vi "Create_Results_Row.vi"() -> (0 "row splitting":string[][](array[string]), 1 "Channel Values":string[](array[string]), 2 "Channel Names":string[](array[string]))   [LabVIEW 2012]
uses:
  Globals/Meas_global.vi
  Globals/Trav_pos_global.vi
  Globals/Dynamic_call_global.ph.vi
  Globals/LDA_meas_global_1.vi
  Acquisition/PWA/PWAtasksGLOBAL.vi
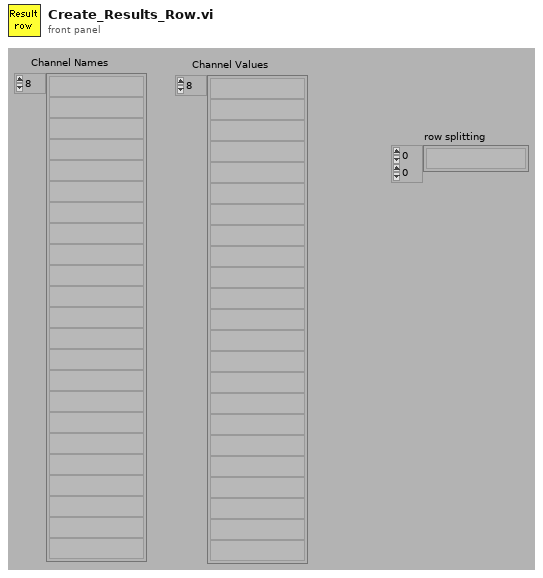
[diagram p1: front panel]
types:
  T1 = typedef "Analysis_info_cluster.ctl" = cluster{"Colour":u32, "Inst type":T2, "Inst name":string, "Symbol":string, "Code name":string, "Extra Info":string, "Inst Array":T3, "Extra Titles":string[], "Extra Values":string[], "U":dbl, "u^2":dbl, "u^3":dbl, "u^4":dbl, "Skew_u":dbl, "Kurt_u":dbl, "Sd Error in Mean":dbl, "% u'/U":dbl, "X":dbl, "Y":dbl, "Z":dbl, "Timescale integral to 25%":dbl, "Sd Error in Variance":dbl, "Calib File":path, "Calib Constants":dbl[], "Output Position":bool, "Full Stats":bool, "Av Sampling Rate":dbl, "Av No of Samples":dbl, "Total Meas Time (s)":dbl, "ADAM Ch Name":string}
  T2 = typedef "Inst_type.ctl" = enum16{"Propeller anemometer", "Raw voltage", "Pressure Transducer", "Pitot-static tube", "Preston tube", "Hot wire", "Cross wire 1", "Cross wire 2", "Generic Linear", "Generic Polynomial", "Generic BackPoly", "Fast FID", "Thermocouple", "Cold wire", "Pulsed Wire", "LDA Vel", "LDA Tran time", "LDA Arr time"}
  T3 = typedef "Instrument_Array.ctl" = enum16{"PWA", "LDA", "Analogue"}
  T4 = typedef "Post_Process.ctl" = enum16{"Take New Data", "Post Process Raw Data File"}
  T5 = typedef "PWA_Data.ctl" = enum16{"No PWA Data", "One Ch PWA"}
  T6 = typedef "Correlation_cluster1.ctl" = cluster{"U inst":string, "uw":dbl, "u^2w":dbl, "uw^2":dbl, "uw/u'w'":dbl, "W inst":string, "uw^3":dbl, "u^3w":dbl, "u^2w^2":dbl, "Index U":i32, "Index W":i32}
  T7 = typedef "Traverse_cluster.ctl" = cluster{"Start X":dbl, "Start Y":dbl, "Start Z":dbl, "End X":dbl, "End Y":dbl, "End Z":dbl, "No. of pts.":i32, "Spacing":T8, "Filename":path, "Tunnel Speed":dbl, "Averaging time (min)":dbl, "Extra Commands":string, "Specific Arguments":string, "Emission Rate (l/min)":dbl, "Trace Gas Concentration (%)":dbl, "Density Ratio":string, "Comments":string, "Row No":i32, "Row Type Selector":T9, "Completion time":string, "Row Duration (mins)":dbl, "No. of Valid pts.":i32, "Meas Setup File":string}
  T8 = typedef "Spacing.ctl" = enum16{"Linear", "Log", "Gauss", "Specified", "N/A"}
  T9 = typedef "Multi_run_mode.ctl" = enum16{"Move Traverse Only", "Set Tunnel Speed Only", "Set Source Only", "Set Measurement Conditions", "Single Measurement", "Vertical Profile", "Lateral Profile", "Longitudinal Profile", "Explore Volume", "Multi-Axis Profile", "Auto Calibrate", "Meas Fast FID Bkgnd", "Check Beam Power", "Scanning Valve Measurement", "Run VI Named:", "Set ADAM Ch", "Wait (minutes)", "Send Message", "Synchronize With:", "Fall Back to this Row", "Turn Off Row Repeating", "Blank Row", "Traverse 3D Volume"}
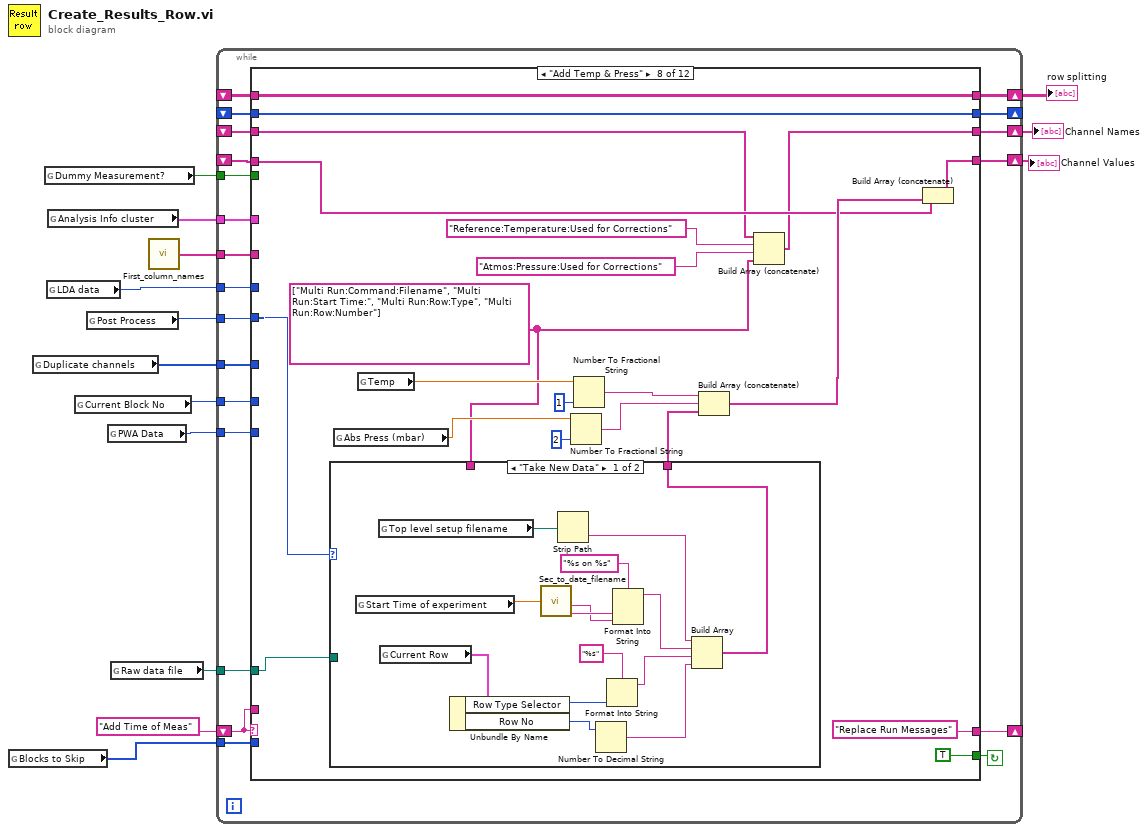
[diagram p0: block diagram]
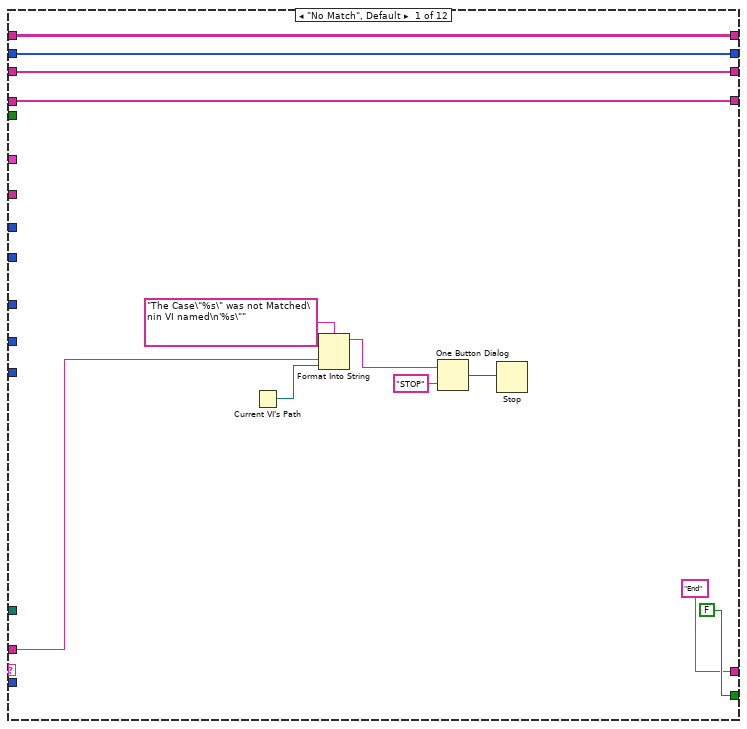
[diagram p2: hidden frame]
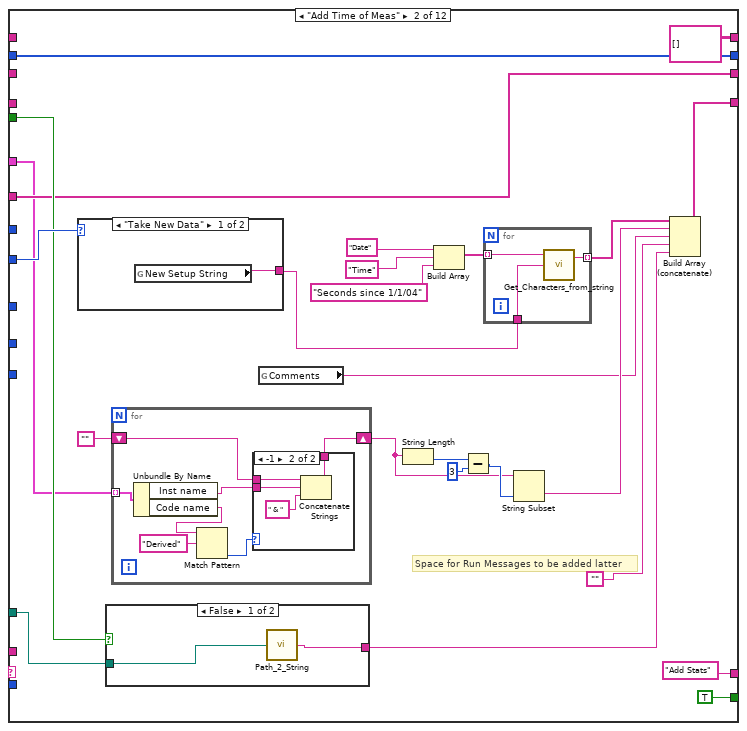
[diagram p3: hidden frame]
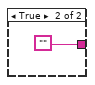
[diagram p4: hidden frame]
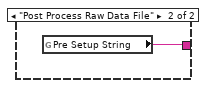
[diagram p6: hidden frame]
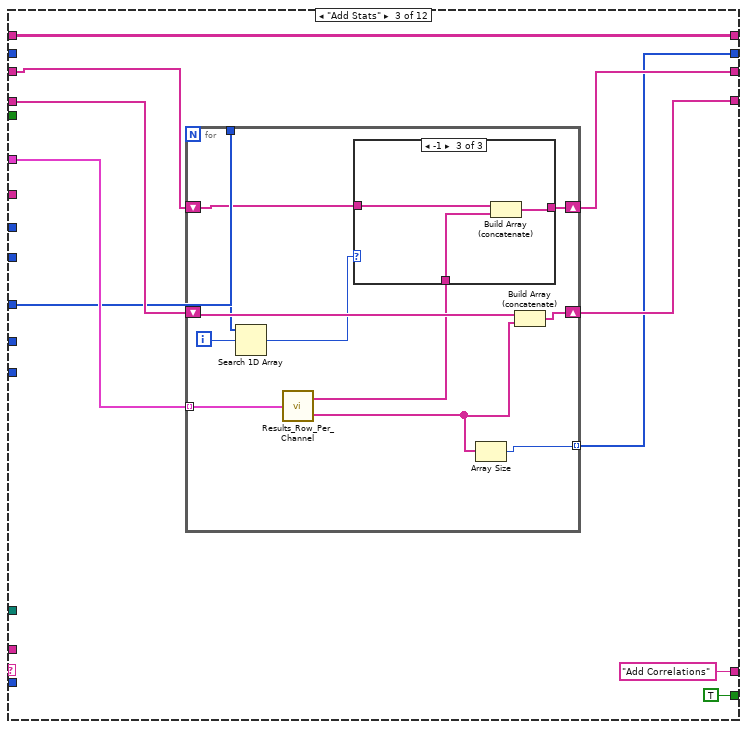
[diagram p7: hidden frame]
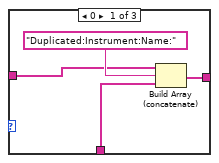
[diagram p8: hidden frame]
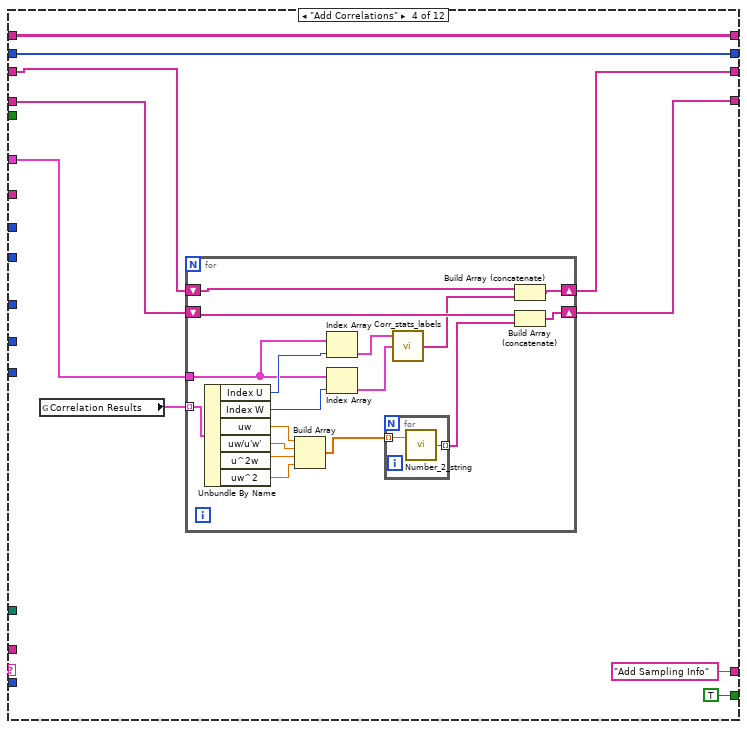
[diagram p10: hidden frame]
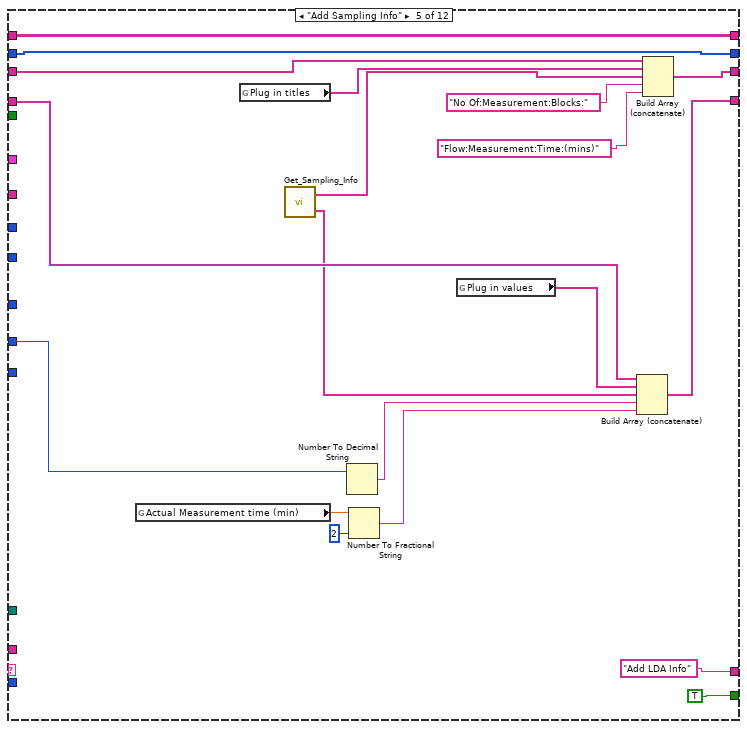
[diagram p11: hidden frame]
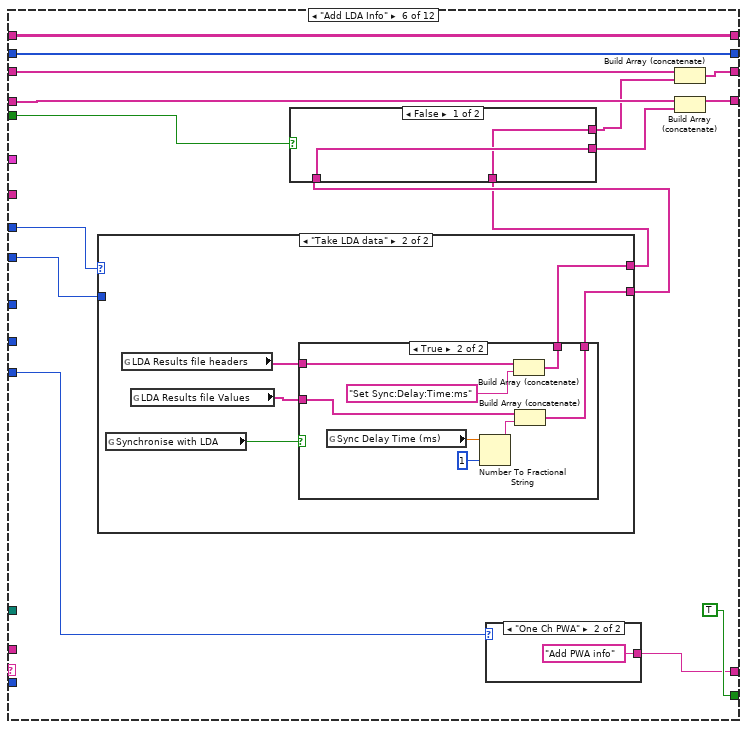
[diagram p12: hidden frame]
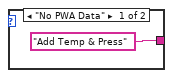
[diagram p13: hidden frame]
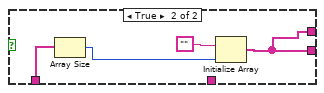
[diagram p14: hidden frame]
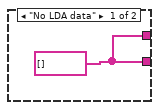
[diagram p15: hidden frame]
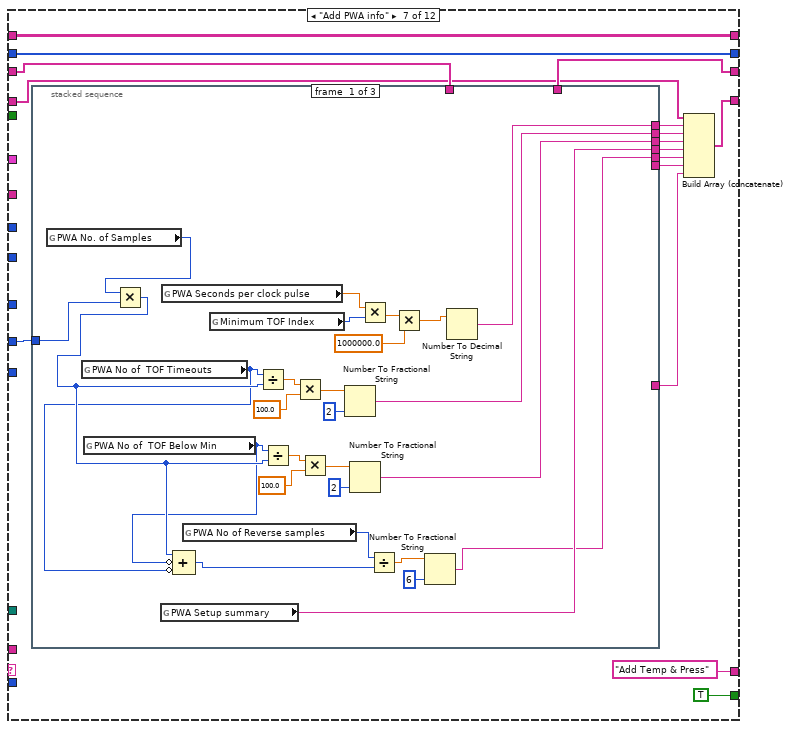
[diagram p17: hidden frame]
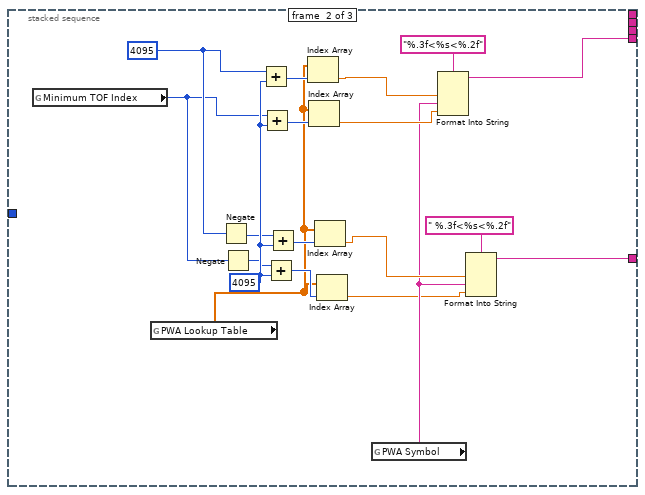
[diagram p18: hidden frame]
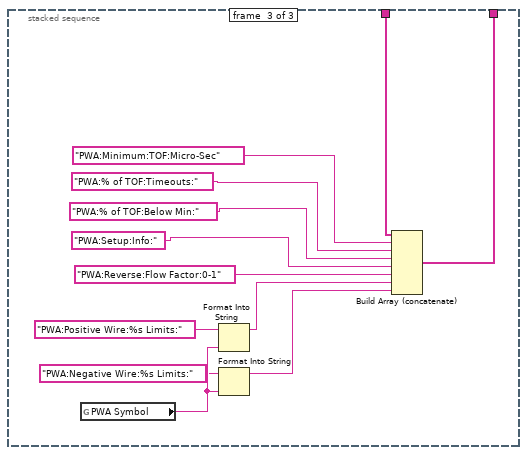
[diagram p19: hidden frame]
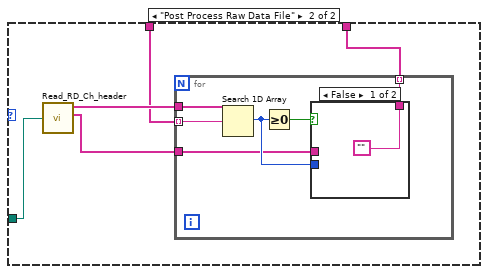
[diagram p20: hidden frame]
diagram:
  n1 = global read "Meas_global.vi" "Blocks to Skip"() -> (w7:i32[])
  n2 = global read "Meas_global.vi" "Duplicate channels"() -> (w3:i32[])
  n3 = global read "Trav_pos_global.vi" "Dummy Measurement?"() -> (w9:bool)
  n4 = global read "Meas_global.vi" "LDA data"() -> (w14:enum16{"No LDA data", "Take LDA data"})
  n5 = global read "Meas_global.vi" "Analysis Info cluster"() -> (w12:T1[])
  n6 = global read "Meas_global.vi" "Current Block No"() -> (w13:i32)
  n7 = global read "Meas_global.vi" "Post Process"() -> (w11:T4)
  n8 = global read "Meas_global.vi" "PWA Data"() -> (w6:T5)
  n9 = global read "Meas_global.vi" "Raw data file"() -> (w5:path)
  n10 = call "First_column_names.vi"() -> ("Array"=w2:string[])
  n11 = while {
    shift-left: _ -> [w28]
    shift-right: [w29] -> w10
    shift-left: "Add Time of Meas" -> [w24]
    shift-right: [w30] -> _
    tunnel: w11 -> [w32]
    tunnel: w12 -> [w33]
    tunnel: w13 -> [w34]
    tunnel: w14 -> [w35]
    tunnel: w9 -> [w27]
    shift-right: [w26] -> w4
    shift-left: _ -> [w25]
    tunnel: w7 -> [w23]
    tunnel: w6 -> [w22]
    tunnel: w5 -> [w21]
    tunnel: w3 -> [w20]
    shift-right: [w19] -> _
    shift-left: _ -> [w18]
    tunnel: w2 -> [w17]
    shift-right: [w16] -> w1
    shift-left: _ -> [w15]
    stop <- w31 continue-if-true
    n12 = case shown="\"Add Temp & Press\"" w24 {
      tunnel: w33 -> [_ w48 w98 w124 _ _ _ _ _ _ _ w445]
      tunnel: w35 -> [_ _ _ _ _ w183 _ _ _ _ _ _]
      tunnel: w34 -> [_ _ _ _ w164 _ w222 _ _ _ _ _]
      tunnel: w32 -> [_ w55 _ _ _ w178 _ w296 _ w381 w423 _]
      tunnel: [FALSE ("Processing last block?") TRUE TRUE ("Processing last block?") TRUE ("Processing last block?") TRUE TRUE ("Processing last block?") TRUE ("Processing last block?") TRUE ("Processing last block?") TRUE ("Processing last block?") TRUE ("Processing last block?") w419 FALSE ("Processing last block?")] -> w31
      tunnel: ["End" "Add Stats" "Add Correlations" ("t") "Add Sampling Info" ("t") "Add LDA Info" w172 "Add Temp & Press" "Replace Run Messages" "Add Plugins" "Add Original Results filename" "Duplicate Chs" "End" ("t")] -> w30
      tunnel: [w39 w71 w99 w128 w163 w184 w223 w304 w350 w376 w428 w438] -> w29
      tunnel: w28 -> [w39 _ w100 w129 w160 w185 w210 w291 w336 w382 w426 w442]
      tunnel: w24 -> [w42 _ _ _ _ _ _ _ _ _ _ _]
      tunnel: w27 -> [_ w54 _ _ _ w182 _ _ w344 _ _ _]
      tunnel: [w38 w50 w101 w130 w158 w175 w213 w285 w342 w372 w416 w437] -> w26
      tunnel: w25 -> [w38 _ w102 w131 w159 w176 w214 w290 w342 w374 w417 w437]
      tunnel: w23 -> [_ _ _ _ _ _ _ _ w338 _ _ _]
      tunnel: w22 -> [_ _ _ _ _ w173 _ _ _ _ _ _]
      tunnel: w21 -> [_ w52 _ _ _ _ _ w295 _ _ _ _]
      tunnel: w20 -> [_ _ w95 _ _ _ _ _ _ _ w421 w441]
      tunnel: [w37 w51 w94 w123 w155 w171 w212 w287 w335 w371 w422 w444] -> w19
      tunnel: w18 -> [w37 w51 _ w123 w155 w171 w212 w287 w335 w371 w422 w444]
      tunnel: w17 -> [_ w50 _ _ _ _ _ _ _ _ _ w443]
      tunnel: [w36 string[][] [] w93 w122 w154 w170 w211 w286 w334 w370 w418 w434] -> w16
      tunnel: w15 -> [w36 _ w93 w122 w154 w170 w211 w286 w334 w370 w418 _]
      frame "No Match", Default {
        n13 = Current VI's Path() -> (path=w43:path)
        n14 = Format Into String(format string="The Case\"%s\" was not Matched\nin VI named\n'%s\"" ("Format String"), w42, w43) -> (resulting string=w46:string)  [unwired: 2 in, 1 out]
        n15 = One Button Dialog(message=w46, button name ("OK")="STOP") -> (true=w44:bool)
        n16 = Stop(stop? (T)=w44) -> ()
      }
      frame "Add Time of Meas" {
        # "Space for Run Messages to be added latter"
        n17 = case shown="\"Take New Data\"" w55 {
          tunnel: [w91 w92] -> w65
          frame "Take New Data" {
            n18 = global read "Meas_global.vi" "New Setup String"() -> (w91:string)
          }
          frame "Post Process Raw Data File" {
            n19 = global read "Meas_global.vi" "Pre Setup String"() -> (w92:string)
          }
        }
        n20 = case shown="False" w54 {
          tunnel: [w74 ""] -> w63
          tunnel: w52 -> [w73 _]
          frame False {
            n21 = call "Path_2_String.vi"("Real Path"=w73) -> ("Path String"=w74:string)
          }
          frame True {
          }
        }
        n22 = for {
          shift-right: [w81] -> w58
          shift-left: "" -> [w82]
          tunnel: w48 -> [w80] mode=indexing
          n23 = Unbundle By Name(w80) -> ("Inst name"=w79:string, "Code name"=w78:string)
          n24 = Match Pattern(string=w78, regular expression="Derived") -> (offset past match=w76:i32)  [unwired: 1 in, 3 out]
          n25 = case shown="-1" w76 {
            tunnel: w82 -> [w83 w87]
            tunnel: [w83 w86] -> w81
            tunnel: w79 -> [_ w84]
            frame 0, Default {
            }
            frame -1 {
              n26 = Concatenate Strings(w87, w84, " & ") -> (w86:string)
            }
          }
        }
        n27 = global read "Meas_global.vi" "Comments"() -> (w53:string)
        n28 = String Length(string=w58) -> (length=w61:i32)
        n29 = Build Array("Date", "Time", "Seconds since 1/1/04") -> (w67:string[])
        n30 = Subtract(x=w61, y=3) -> (x-y=w59:i32)
        n31 = for {
          tunnel: w67 -> [w90] mode=indexing
          tunnel: w65 -> [w89]
          tunnel: [w88] -> w66 mode=indexing
          n32 = call "Get_Characters_from_string.vi"("Input string"=w89, "Variable name"=w90) -> ("Value"=w88:string)  [unwired: 1 in, 1 out]
        }
        n33 = String Subset(string=w58, length (rest)=w59) -> (substring=w56:string)  [unwired: 1 out]
        n34 = Build Array (concatenate)(w66, w56, w53, "", w63) -> (w71:string[])
      }
      frame "Add Stats" {
        n35 = for {
          shift-right: [w110] -> w101
          shift-left: w102 -> [w112]
          shift-right: [w113] -> w99
          shift-left: w100 -> [w111]
          tunnel: w98 -> [w109] mode=indexing
          tunnel: [w106] -> w94 mode=indexing
          tunnel: w95 -> [w104]
          i -> [w105]
          n36 = Search 1D Array(1D array=w104, element=w105) -> (index of element=w103:i32)  [unwired: 1 out]
          n37 = call "Results_Row_Per_Channel.vi"("Analysis_info_cluster"=w109) -> ("Channel Names"=w108:string[], "Channel Values"=w107:string[])
          n38 = case shown="-1" w103 {
            tunnel: w112 -> [w116 w118 w121]
            tunnel: [w114 w118 w120] -> w110
            tunnel: w108 -> [w115 _ w119]
            frame 0 {
              n39 = Build Array (concatenate)(w116, "Duplicated:Instrument:Name:", w115) -> (w114:string[])
            }
            frame 1, Default {
            }
            frame -1 {
              n40 = Build Array (concatenate)(w121, w119) -> (w120:string[])
            }
          }
          n41 = Array Size(array=w107) -> (size(s)=w106:i32)
          n42 = Build Array (concatenate)(w111, w107) -> (w113:string[])
        }
      }
      frame "Add Correlations" {
        n43 = global read "Meas_global.vi" "Correlation Results"() -> (w125:T6[])
        n44 = for {
          shift-right: [w145] -> w130
          shift-left: w131 -> [w147]
          shift-right: [w148] -> w128
          shift-left: w129 -> [w146]
          tunnel: w125 -> [w144] mode=indexing
          tunnel: w124 -> [w141]
          n45 = Unbundle By Name(w144) -> ("Index U"=w143:i32, "Index W"=w142:i32, "uw"=w137:dbl, "uw/u'w'"=w136:dbl, "u^2w"=w135:dbl, "uw^2"=w134:dbl)
          n46 = Build Array(w137, w136, w135, w134) -> (w133:dbl[])
          n47 = Index Array(array=w141, index=w143) -> (element=w140:T1)
          n48 = Index Array(array=w141, index=w142) -> (element=w139:T1)
          n49 = for {
            tunnel: w133 -> [w150] mode=indexing
            tunnel: [w149] -> w132 mode=indexing
            n50 = call "Number_2_string.vi"("number"=w150) -> ("String"=w149:string)  [unwired: 1 in]
          }
          n51 = call "Corr_stats_labels.vi"("Inst 2 Units"=w139, "Inst 1 Units"=w140) -> ("Output"=w138:string[])  [unwired: 1 in]
          n52 = Build Array (concatenate)(w147, w138) -> (w145:string[])
          n53 = Build Array (concatenate)(w146, w132) -> (w148:string[])
        }
      }
      frame "Add Sampling Info" {
        n54 = global read "Meas_global.vi" "Actual Measurement time (min)"() -> (w165:dbl)
        n55 = global read "Dynamic_call_global.ph.vi" "Plug in titles"() -> (w157:string[])
        n56 = call "Get_Sampling_Info.vi"() -> ("Channel Values"=w152:string[], "Channel Names"=w153:string[])  [unwired: 2 in]
        n57 = Number To Decimal String(number=w164) -> (decimal integer string=w162:string)  [unwired: 1 out]
        n58 = Number To Fractional String(number=w165, precision (6)=i16 2) -> (F-format string=w167:string)  [unwired: 2 out]
        n59 = global read "Dynamic_call_global.ph.vi" "Plug in values"() -> (w161:string[])
        n60 = Build Array (concatenate)(w160, w161, w152, w162, w167) -> (w163:string[])
        n61 = Build Array (concatenate)(w159, w157, w153, "No Of:Measurement:Blocks:", "Flow:Measurement:Time:(mins)") -> (w158:string[])
      }
      frame "Add LDA Info" {
        n62 = case shown="\"Take LDA data\"" w183 {
          tunnel: w178 -> [_ _]
          tunnel: [w194 w195] -> w179
          tunnel: [w194 w197] -> w177
          frame "No LDA data" {
            w194 = string[] []
          }
          frame "Take LDA data" {
            n63 = global read "Meas_global.vi" "Synchronise with LDA"() -> (w199:bool)
            n64 = global read "LDA_meas_global_1.vi" "LDA Results file headers"() -> (w198:string[])
            n65 = global read "LDA_meas_global_1.vi" "LDA Results file Values"() -> (w196:string[])
            n66 = case shown="True" w199 {
              tunnel: w198 -> [w201 w207]
              tunnel: [w201 w205] -> w197
              tunnel: w196 -> [w200 w204]
              tunnel: [w200 w202] -> w195
              frame False {
              }
              frame True {
                n67 = global read "LDA_meas_global_1.vi" "Sync Delay Time (ms)"() -> (w208:dbl)
                n68 = Number To Fractional String(number=w208, precision (6)=i16 1) -> (F-format string=w203:string)  [unwired: 2 out]
                n69 = Build Array (concatenate)(w207, "Set Sync:Delay:Time:ms" ("Input Element")) -> (w205:string[])
                n70 = Build Array (concatenate)(w204, w203) -> (w202:string[])
              }
            }
          }
        }
        n71 = case shown="False" w182 {
          tunnel: [w189 w190] -> w181
          tunnel: w179 -> [w189 w193]
          tunnel: [w188 w190] -> w174
          tunnel: w177 -> [w188 _]
          frame False {
          }
          frame True {
            n72 = Array Size(array=w193) -> (size(s)=w192:i32)
            n73 = Initialize Array("", w192) -> (w190:string[])
          }
        }
        n74 = case shown="\"One Ch PWA\"" w173 {
          tunnel: ["Add Temp & Press" "Add PWA info"] -> w172
          frame "No PWA Data" {
          }
          frame "One Ch PWA" {
          }
        }
        n75 = Build Array (concatenate)(w176, w174) -> (w175:string[])
        n76 = Build Array (concatenate)(w185, w181) -> (w184:string[])
      }
      frame "Add PWA info" {
        n77 = stacked-sequence {
          tunnel: w222 -> [w251 _ _]
          tunnel: [w246 _ _] -> w221
          tunnel: [w241 _ _] -> w220
          tunnel: [w240 _ _] -> w219
          tunnel: [_ w254 _] -> w218
          tunnel: [_ w253 _] -> w217
          tunnel: [w234 _ _] -> w216
          tunnel: [w226 _ _] -> w215
          tunnel: w214 -> [_ _ w273]
          tunnel: [_ _ w272] -> w213
          frame #0 {
            n78 = global read "PWAtasksGLOBAL.vi" "PWA No. of Samples"() -> (w252:i32)
            n79 = global read "PWAtasksGLOBAL.vi" "PWA No of  TOF Timeouts"() -> (w231:i32)
            n80 = global read "PWAtasksGLOBAL.vi" "PWA No of  TOF Below Min"() -> (w232:i32)
            n81 = Multiply(x=w252, y=w251) -> (x*y=w233:i32)
            n82 = global read "PWAtasksGLOBAL.vi" "PWA Setup summary"() -> (w240:string)
            n83 = global read "PWAtasksGLOBAL.vi" "PWA Seconds per clock pulse"() -> (w238:dbl)
            n84 = Compound Arithmetic op=ADD(w233, invert w232, invert w231) -> (w229:i32)
            n85 = global read "PWAtasksGLOBAL.vi" "PWA No of Reverse samples"() -> (w230:i32)
            n86 = global read "PWAtasksGLOBAL.vi" "Minimum TOF Index"() -> (w239:i16)
            n87 = Divide(x=w231, y=w233) -> (x/y=w250:dbl)
            n88 = Divide(x=w232, y=w233) -> (x/y=w242:dbl)
            n89 = Multiply(x=w250, y=100.0) -> (x*y=w247:dbl)
            n90 = Multiply(x=w242, y=100.0) -> (x*y=w245:dbl)
            n91 = Number To Fractional String(number=w247, precision (6)=i16 2) -> (F-format string=w246:string)  [unwired: 2 out]
            n92 = Number To Fractional String(number=w245, precision (6)=i16 2) -> (F-format string=w241:string)  [unwired: 2 out]
            n93 = Multiply(x=w238, y=w239) -> (x*y=w237:dbl)
            n94 = Divide(x=w230, y=w229) -> (x/y=w227:dbl)
            n95 = Multiply(x=w237, y=1000000.0) -> (x*y=w235:dbl)
            n96 = Number To Fractional String(number=w227, precision (6)=i16 6) -> (F-format string=w226:string)  [unwired: 2 out]
            n97 = Number To Decimal String(number=w235) -> (decimal integer string=w234:string)  [unwired: 1 out]
          }
          frame #1 {
            w267 = 4095
            w263 = 4095
            n98 = global read "PWAtasksGLOBAL.vi" "Minimum TOF Index"() -> (w262:i16)
            n99 = global read "PWAtasksGLOBAL.vi" "PWA Lookup Table"() -> (w266:dbl[])
            n100 = Negate(x=w263) -> (-x=w265:i32)
            n101 = Negate(x=w262) -> (-x=w264:i16)
            n102 = Add(x=w263, y=w267) -> (x+y=w268:i32)
            n103 = Add(x=w262, y=w267) -> (x+y=w269:i32)
            n104 = Add(x=w264, y=w267) -> (x+y=w271:i32)
            n105 = Add(x=w265, y=w267) -> (x+y=w270:i32)
            n106 = Index Array(array=w266, index=w268) -> (element=w261:dbl)
            n107 = Index Array(array=w266, index=w269) -> (element=w260:dbl)
            n108 = Index Array(array=w266, index=w270) -> (element=w257:dbl)
            n109 = Index Array(array=w266, index=w271) -> (element=w255:dbl)
            n110 = global read "PWAtasksGLOBAL.vi" "PWA Symbol"() -> (w256:string)
            n111 = Format Into String(format string="%.3f<%s<%.2f", w261, w256, w260) -> (resulting string=w254:string)  [unwired: 2 in, 1 out]
            n112 = Format Into String(format string=" %.3f<%s<%.2f", w257, w256, w255) -> (resulting string=w253:string)  [unwired: 2 in, 1 out]
          }
          frame #2 {
            n113 = global read "PWAtasksGLOBAL.vi" "PWA Symbol"() -> (w276:string)
            n114 = Format Into String(format string="PWA:Positive Wire:%s Limits:", w276) -> (resulting string=w280:string)  [unwired: 2 in, 1 out]
            n115 = Format Into String(format string="PWA:Negative Wire:%s Limits:", w276) -> (resulting string=w281:string)  [unwired: 2 in, 1 out]
            n116 = Build Array (concatenate)(w273, "PWA:Minimum:TOF:Micro-Sec", "PWA:% of TOF:Timeouts:", "PWA:% of TOF:Below Min:", "PWA:Setup:Info:", "PWA:Reverse:Flow Factor:0-1", w280, w281) -> (w272:string[])
          }
        }
        n117 = Build Array (concatenate)(w210, w216, w221, w220, w219, w215, w218, w217) -> (w223:string[])
      }
      frame "Add Temp & Press" {
        w284 = string[] ["Multi Run:Command:Filename", "Multi Run:Start Time:", "Multi Run:Row:Type", "Multi Run:Row:Number"] ("appended array")
        n118 = case shown="\"Take New Data\"" w296 {
          tunnel: [w307 w320] -> w297
          tunnel: w295 -> [_ w323]
          tunnel: w284 -> [_ w319]
          frame "Take New Data" {
            n119 = global read "Meas_global.vi" "Start Time of experiment"() -> (w318:dbl)
            n120 = global read "Trav_pos_global.vi" "Top level setup filename"() -> (w306:path)
            n121 = global read "Trav_pos_global.vi" "Current Row"() -> (w313:T7)
            n122 = Unbundle By Name(w313) -> ("Row Type Selector"=w312:T9, "Row No"=w309:i32)
            n123 = call "Sec_to_date_filename.vi"("seconds"=w318) -> ("Day"=w316:string, "Time"=w317:string)  [unwired: 2 out]
            n124 = Strip Path(path=w306) -> (name=w305:string)  [unwired: 1 out]
            n125 = Number To Decimal String(number=w309) -> (decimal integer string=w308:string)  [unwired: 1 in]
            n126 = Format Into String(format string="%s", w312) -> (resulting string=w310:string)  [unwired: 2 in, 1 out]
            n127 = Format Into String(format string="%s on %s", w317, w316) -> (resulting string=w314:string)  [unwired: 2 in, 1 out]
            n128 = Build Array(w305, w314, w310, w308) -> (w307:string[])
          }
          frame "Post Process Raw Data File" {
            n129 = call "Read_RD_Ch_header.vi"("Raw data file"=w323) -> ("Ch Name Out"=w322:string[], "Ch Values"=w321:string[])  [unwired: 2 out]
            n130 = for {
              tunnel: w322 -> [w329]
              tunnel: w321 -> [w326]
              tunnel: [w325] -> w320 mode=indexing
              tunnel: w319 -> [w324] mode=indexing
              n131 = Search 1D Array(1D array=w329, element=w324) -> (index of element=w327:i32)  [unwired: 1 out]
              n132 = Greater Or Equal To 0?(x=w327) -> (x >= 0?=w328:bool)
              n133 = case shown="False" w328 {
                tunnel: w327 -> [_ w333]
                tunnel: w326 -> [_ w332]
                tunnel: ["" w331] -> w325
                frame False {
                }
                frame True {
                  n134 = Index Array(array=w332, index=w333) -> (element=w331:string)
                }
              }
            }
          }
        }
        n135 = global read "Meas_global.vi" "Abs Press (mbar)"() -> (w302:dbl)
        n136 = global read "Meas_global.vi" "Temp"() -> (w298:dbl)
        n137 = Number To Fractional String(number=w302, precision (6)=i16 2) -> (F-format string=w303:string)  [unwired: 2 out]
        n138 = Number To Fractional String(number=w298, precision (6)=i16 1) -> (F-format string=w300:string)  [unwired: 2 out]
        n139 = Build Array (concatenate)(w300, w303, w297) -> (w292:string[])
        n140 = Build Array (concatenate)(w290, "Reference:Temperature:Used for Corrections", "Atmos:Pressure:Used for Corrections", w284) -> (w285:string[])
        n141 = Build Array (concatenate)(w291, w292) -> (w304:string[])
      }
      frame "Replace Run Messages" {
        n142 = Array Size(array=w338) -> (size(s)=w339:i32)
        n143 = global read "Meas_global.vi" "BSA data rate string"() -> (w352:string)
        n144 = global read "Meas_global.vi" "Over/Under string"() -> (w354:string)
        n145 = Equal To 0?(x=w339) -> (x = 0?=w337:bool)
        n146 = global read "Meas_global.vi" "Extra Comments"() -> (w353:string)
        n147 = Concatenate Strings(w352, w354, w353) -> (w351:string)
        n148 = call "Remove_unprintable_Char.vi"("Input String"=w351) -> ("Output String"=w341:string)
        n149 = case shown="False" w337 {
          tunnel: w338 -> [w360 _]
          tunnel: w341 -> [w356 w365]
          tunnel: [w355 w365] -> w340
          frame False {
            n150 = for {
              shift-right: [w362] -> w358
              shift-left: "Blocks " -> [w364]
              tunnel: w360 -> [w363] mode=indexing
              n151 = Format Into String(format string="%d; ", initial string=w364, w363) -> (resulting string=w362:string)  [unwired: 1 in, 1 out]
            }
            n152 = Concatenate Strings(w356, w358, "have been skipped. " ("string")) -> (w355:string)
          }
          frame True {
          }
        }
        n153 = case shown="False" w344 {
          tunnel: [w366 "Dummy Measurement"] -> w343
          tunnel: w340 -> [w366 _]
          frame False {
          }
          frame True {
          }
        }
        n154 = call "First_column_names.vi"() -> ("Array"=w347:string[])
        n155 = Search 1D Array(1D array=w347, element="Run:Messages::") -> (index of element=w346:i32)  [unwired: 1 out]
        n156 = Replace Array Subset(array=w336, new element=w343, index=w346) -> (w350:string[])
      }
      frame "Add Plugins" {
        n157 = case shown="\"Take New Data\"" w381 {
          tunnel: ["Take New Data" "Post Process"] -> w380
          frame "Take New Data" {
          }
          frame "Post Process Raw Data File" {
          }
        }
        n158 = global read "Meas_global.vi" "Acquisition vi to Run"() -> (w368:string)
        n159 = Build Array (concatenate)(w374, "Prog Post:Process:Mode" ("Input Element"), "Acquisition:PlugIn:Used" ("Input Element")) -> (w373:string[])
        n160 = Build Array (concatenate)(w382, w380, w368) -> (w377:string[])
        n161 = for {
          N: 3 -> [_]
          shift-right: [w389] -> w376
          shift-left: w377 -> [w390]
          shift-right: [w385] -> w372
          shift-left: w373 -> [w386]
          i -> [w393]
          n162 = case shown="0, Default" w393 {
            tunnel: [w404 w406 w408] -> w387
            tunnel: ["Initial:PlugIns:Used" ("Input Element") "Per Block:PlugIns:Used" ("Input Element") "Final:PlugIns:Used" ("Input Element")] -> w384
            frame 0, Default {
              n163 = global read "Dynamic_call_global.ph.vi" "Initial Plug Ins"() -> (w404:string[])
            }
            frame 1 {
              n164 = global read "Dynamic_call_global.ph.vi" "Per Block Plug Ins"() -> (w406:string[])
            }
            frame 2 {
              n165 = global read "Dynamic_call_global.ph.vi" "Final Plug Ins"() -> (w408:string[])
            }
          }
          n166 = Array Size(array=w387) -> (size(s)=w392:i32)
          n167 = for {
            tunnel: w387 -> [w409] mode=indexing
            shift-right: [w410] -> w388
            shift-left: "" -> [w412]
            n168 = Concatenate Strings(w412, w409, ";" ("string")) -> (w410:string)
          }
          n169 = Greater Than 0?(x=w392) -> (x > 0?=w391:bool)
          n170 = case shown="True" w391 {
            tunnel: w390 -> [w396 w402]
            tunnel: [w396 w401] -> w389
            tunnel: w388 -> [_ w400]
            tunnel: w386 -> [w395 w399]
            tunnel: [w395 w398] -> w385
            tunnel: w384 -> [_ w397]
            frame False {
            }
            frame True {
              n171 = Build Array (concatenate)(w402, w400) -> (w401:string[])
              n172 = Build Array (concatenate)(w399, w397) -> (w398:string[])
            }
          }
        }
      }
      frame "Add Original Results filename" {
        n173 = case shown="\"Post Process Raw Data File\"" w423 {
          tunnel: [w429 w433] -> w425
          frame "Post Process Raw Data File" {
            n174 = global read "Meas_global.vi" "Pre Setup String"() -> (w432:string)
            n175 = call "Get_Characters_from_string.vi"("Input string"=w432, "Variable name"="Results filename") -> ("Value"=w430:string)  [unwired: 1 in, 1 out]
            n176 = call "String_to_Pathname.vi"("Input String"=w430) -> ("path"=w429:path)
          }
          frame "Take New Data" {
            n177 = global read "Meas_global.vi" "Results file"() -> (w433:path)
          }
        }
        n178 = Array Size(array=w421) -> (size(s)=w420:i32)
        n179 = Not Equal To 0?(x=w420) -> (x != 0?=w419:bool)
        n180 = Strip Path(path=w425) -> (name=w424:string)  [unwired: 1 out]
        n181 = Build Array (concatenate)(w417, "Original:Results:Filename") -> (w416:string[])
        n182 = Build Array (concatenate)(w426, w424) -> (w428:string[])
      }
      frame "Duplicate Chs" {
        n183 = Array Size(array=w443) -> (size(s)=w447:i32)
        n184 = Split 1D Array(array=w442, index=w447) -> (first subarray=w448:string[], second subarray=w450:string[])
        n185 = Add Array Elements(numeric array=w444) -> (sum=w449:i32)
        n186 = Array Subset(array=w450, index=w449) -> (w439:string[])  [unwired: 1 in]
        n187 = for {
          shift-right: [w463] -> w440
          shift-left: w448 -> [w464]
          tunnel: w444 -> [w462] mode=indexing
          tunnel: w450 -> [w465]
          shift-right: [w461] -> _
          shift-left: 0 -> [w460]
          tunnel: w441 -> [w458]
          shift-right: [w456] -> w434
          shift-left: string[][] [] -> [w455]
          tunnel: w445 -> [w452] mode=indexing
          i -> [w454]
          n188 = Unbundle By Name(w452) -> ("Inst name"=w453:string)
          n189 = Search 1D Array(1D array=w458, element=w454) -> (index of element=w457:i32)  [unwired: 1 out]
          n190 = Array Subset(array=w465, index=w460, length=w462) -> (w459:string[])
          n191 = Add(x=w462, y=w460) -> (x+y=w461:i32)
          n192 = case shown="0" w457 {
            tunnel: w464 -> [w469 w476 w478]
            tunnel: [w468 w477 w478] -> w463
            tunnel: w459 -> [w467 w473 w482]
            tunnel: w453 -> [_ w474 w483]
            tunnel: [w466 w471 w480] -> w456
            tunnel: w455 -> [w466 w470 w479]
            frame -1 {
              n193 = Build Array (concatenate)(w469, w467) -> (w468:string[])
            }
            frame 0 {
              n194 = Build Array (concatenate)(w474, w473) -> (w472:string[])
              n195 = Build Array (concatenate)(w476, "Instrument_name_place_holder", w473) -> (w477:string[])
              n196 = Build Array (concatenate)(w470, w472) -> (w471:string[][])
            }
            frame 1, Default {
              n197 = Build Array (concatenate)(w483, w482) -> (w481:string[])
              n198 = Build Array (concatenate)(w479, w481) -> (w480:string[][])
            }
          }
        }
        n199 = Build Array (concatenate)(w440, w439) -> (w438:string[])
      }
    }
  }
  "Channel Values" <- w10
  "Channel Names" <- w4
  "row splitting" <- w1
